vi "상태24.vi"(7 "FGV":enum16{"Set", "Get"}(ring), 8 "error in":errorcluster, 11 "상태":enum16{"초기화", "대기", "재생", "일지정지", "취소"}(ring)) -> (0 "error out":errorcluster, 2 "상태 출력":enum16{"초기화", "대기", "재생", "일지정지", "취소"}(ring))   [LabVIEW 2020]
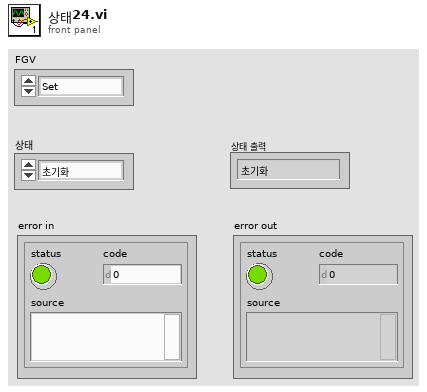
[diagram p1: front panel]
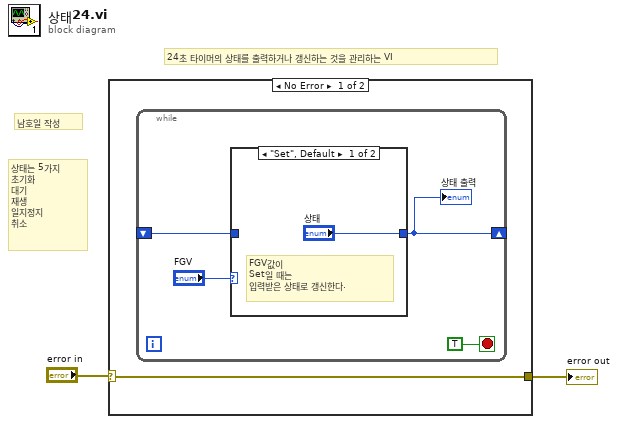
[diagram p0: block diagram]
diagram:
  # "상태는 5가지 \n초기화\n대기\n재생\n일지정지\n취소"
  # "남호일 작성"
  # "24초 타이머의 상태를 출력하거나 갱신하는 것을 관리하는 VI"
  n1 = case shown="No Error" "error in" {
    selector: "error in" -> [w3 w10]
    tunnel: [w3 w10] -> w1
    frame No Error {
      n2 = while {
        shift-right: [w5] -> _
        shift-left: _ -> [w4]
        stop <- TRUE stop-if-true
        n3 = case shown="\"Set\", Default" "FGV" {
          tunnel: ["상태" w9] -> w5
          tunnel: w4 -> [_ w9]
          frame "Set", Default {
            # "FGV값이 \nSet일 때는\n입력받은 상태로 갱신한다."
          }
          frame "Get" {
            # "FGV값이 \nGet일 때는 \n현재 상태를 출력한다."
          }
        }
        "상태 출력" <- w5
      }
    }
    frame Error {
    }
  }
  "error out" <- w1
